vi "bool82bool.vi"(1 "bool8 in":u8) -> (0 "bool out":bool)   [LabVIEW 2018, in "LibTiePie.lvlib"]
uses:
  LibTiePie.lvlib
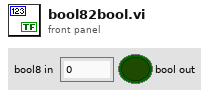
[diagram p1: front panel]
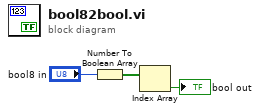
[diagram p0: block diagram]
diagram:
  n1 = Number To Boolean Array(number="bool8 in") -> (Boolean array=w2:bool[])
  n2 = Index Array(array=w2) -> (element=→"bool out":bool)  [unwired: 1 in]
